vi "RX ADU.vi"(8 "error in (no error)":errorcluster, 9 "RX Data":string, 11 "MB_ADU_TCP in":refnum<class "MB_ADU_TCP.lvclass">) -> (0 "error out":errorcluster, 1 "PDU_resp":T1={"Function Code"=1, "Data"=[], "RTU_DataBytes"=0}, 3 "MB_ADU_TCP out":refnum<class "MB_ADU_TCP.lvclass">)   [LabVIEW 2016, in "MB Master.lvlib" / "MB_ADU_TCP.lvclass"]
doc: "Defines the receive procedure for a Modbus TCP ADU. The received PDU is written to PDU_resp."
uses:
  MB_ADU_TCP.lvclass
  MB_PDU/MB_PDU_Cluster.ctl
  MB Master.lvlib
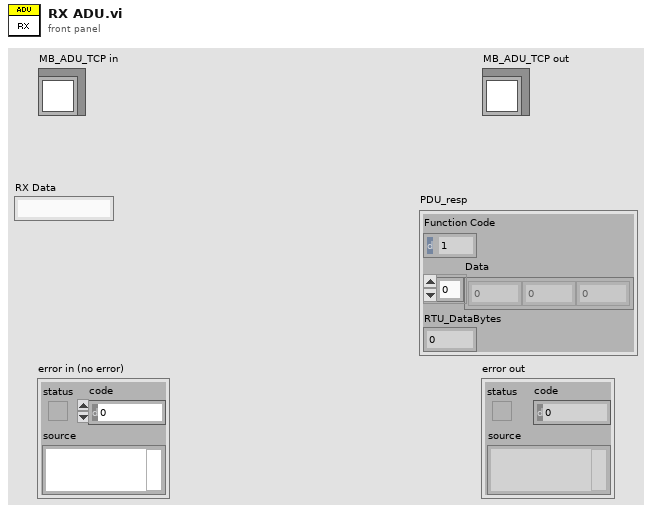
[diagram p1: front panel]
types:
  T1 = typedef "MB Master.lvlib/MB_PDU_Cluster.ctl" = cluster{"Function Code":u8, "Data":u8[], "RTU_DataBytes":i32}
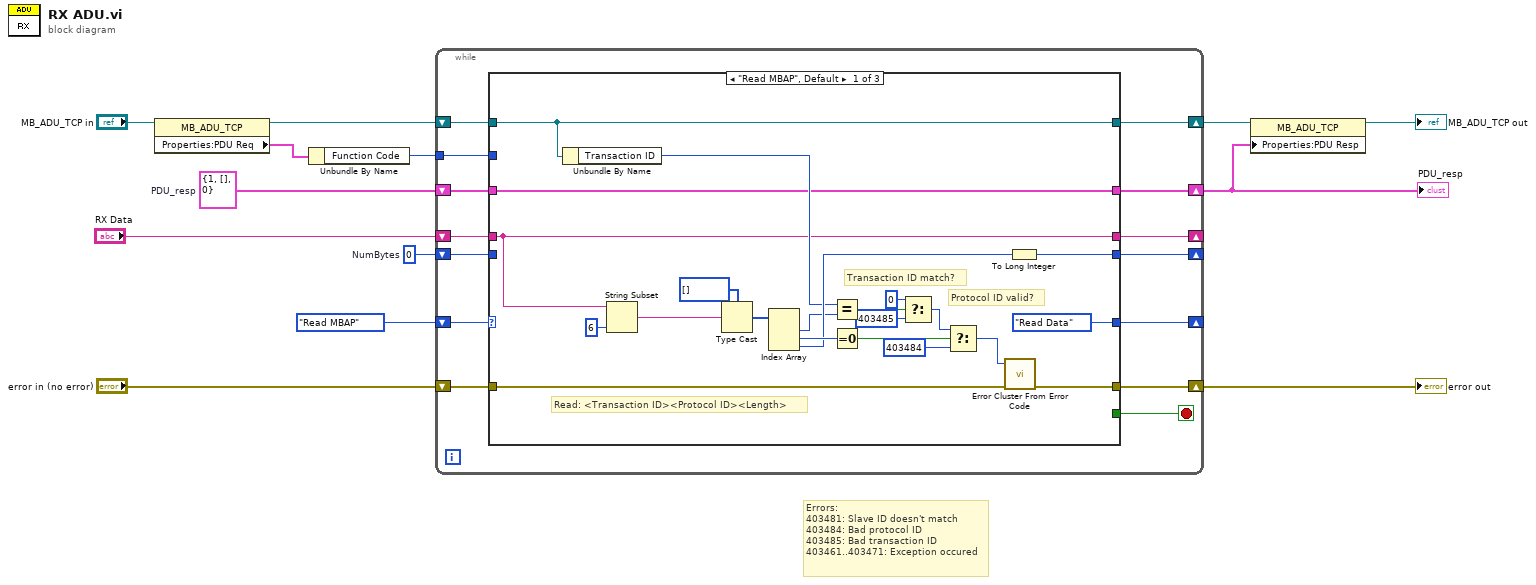
[diagram p0: block diagram]
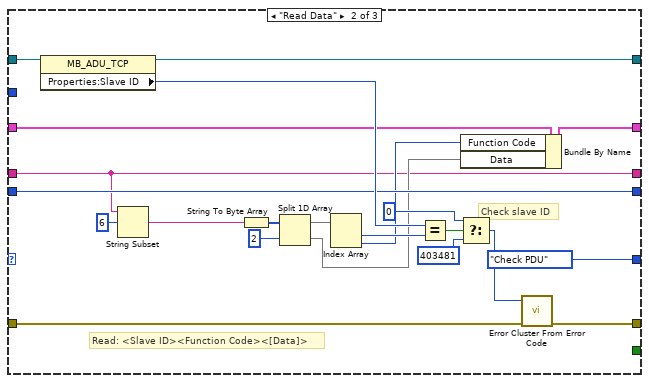
[diagram p2: hidden frame]
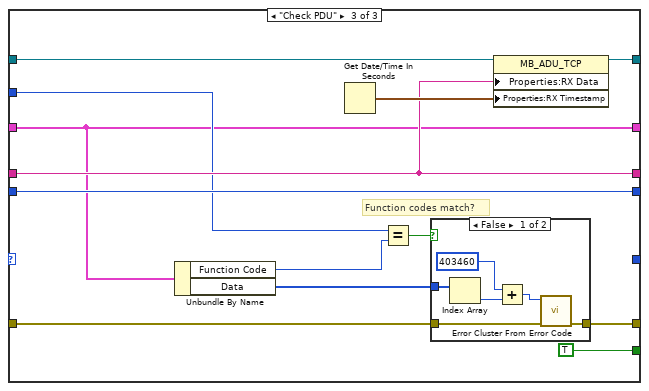
[diagram p3: hidden frame]
diagram:
  w7 = T1 {"Function Code"=1, "Data"=[], "RTU_DataBytes"=0}  # PDU_resp
  w10 = 0  # NumBytes
  # "Errors:\n403481: Slave ID doesn't match\n403484: Bad protocol ID\n403485: Bad transaction ID \n403461..403471: Exception occured"
  n1 = property class="MB_ADU_TCP"(reference="MB_ADU_TCP in") -> (reference out=w2:refnum<class "MB_ADU_TCP.lvclass">, "Properties:PDU Req"=w1:T1)  [unwired: 1 in, 1 out]
  n2 = Unbundle By Name(w1) -> ("Function Code"=w8:u8)
  n3 = while {
    shift-right: [w26] -> w11
    shift-left: "error in (no error)" -> [w25]
    shift-right: [w23] -> _
    shift-left: w10 -> [w20]
    shift-right: [w22] -> _
    shift-left: "RX Data" -> [w21]
    shift-right: [w18] -> w6
    shift-left: w2 -> [w19]
    shift-right: [w17] -> _
    shift-left: enum16{"Read MBAP", "Read Data", "Check PDU"}."Read MBAP" -> [w27]
    tunnel: w8 -> [w16]
    shift-right: [w14] -> w4
    shift-left: w7 -> [w15]
    stop <- w24 stop-if-true
    n4 = case shown="\"Read MBAP\", Default" w27 {
      tunnel: [w42 w61 w77] -> w26
      tunnel: w25 -> [w31 w51 w78]
      tunnel: [_ _ TRUE ("status")] -> w24
      tunnel: [w45 w59 w81] -> w23
      tunnel: [w29 w50 w82] -> w22
      tunnel: w21 -> [w29 w50 w82]
      tunnel: w20 -> [_ w59 w81]
      tunnel: w19 -> [w39 w60 w72]
      tunnel: [w39 w58 w83] -> w18
      tunnel: [enum16{"Read MBAP", "Read Data", "Check PDU"}."Read Data" enum16{"Read MBAP", "Read Data", "Check PDU"}."Check PDU" _] -> w17
      tunnel: w16 -> [_ _ w76]
      tunnel: w15 -> [w32 w57 w75]
      tunnel: [w32 w54 w75] -> w14
      frame "Read MBAP", Default {
        # "Transaction ID match?"
        # "Protocol ID valid?"
        # "Read: <Transaction ID><Protocol ID><Length>"
        n5 = Unbundle By Name(w39) -> ("Transaction ID"=w37:u16)
        n6 = String Subset(string=w29, length (rest)=6 ("length (rest)")) -> (substring=w28:string)  [unwired: 1 in]
        n7 = Type Cast(type=u16[] [], x=w28) -> (*(type *) &x=w48:u16[])
        n8 = Index Array(array=w48) -> (element #1=w38:u16, element #2=w47:u16, element #3=w46:u16)  [unwired: 3 in]
        n9 = Equal?(x=w37, y=w38) -> (x = y?=w36:bool)
        n10 = Equal To 0?(x=w47) -> (x = 0?=w44:bool)
        n11 = Select(t=0, s=w36, f=403485) -> (s? t:f=w34:i32)
        n12 = Select(t=w34, s=w44, f=403484) -> (s? t:f=w41:i32)
        n13 = call <vilib>:"Error Cluster From Error Code.vi"("error in (no error)"=w31, "error code (0)"=w41) -> ("error out"=w42:errorcluster)  [unwired: 7 in]
        n14 = To Long Integer(number=w46) -> (32bit integer=w45:i32)
      }
      frame "Read Data" {
        # "Check slave ID"
        # "Read: <Slave ID><Function Code><[Data]>"
        n15 = property class="MB_ADU_TCP"(reference=w60) -> (reference out=w58:refnum<class "MB_ADU_TCP.lvclass">, "Properties:Slave ID"=w66:u8)  [unwired: 1 in, 1 out]
        n16 = String Subset(string=w50, offset (0)=6) -> (substring=w52:string)  [unwired: 1 in]
        n17 = String To Byte Array(string=w52) -> (unsigned byte array=w71:u8[])
        n18 = Split 1D Array(array=w71, index=2) -> (first subarray=w70:u8[], second subarray=w55:u8[])
        n19 = Index Array(array=w70) -> (element #1=w67:u8, element #2=w56:u8)  [unwired: 2 in]
        n20 = Equal?(x=w66, y=w67) -> (x = y?=w65:bool)
        n21 = Bundle By Name(cluster=w57, "Function Code"=w56, "Data"=w55) -> (w54:T1)
        n22 = Select(t=0, s=w65, f=403481) -> (s? t:f=w62:i32)
        n23 = call <vilib>:"Error Cluster From Error Code.vi"("error in (no error)"=w51, "error code (0)"=w62) -> ("error out"=w61:errorcluster)  [unwired: 7 in]
      }
      frame "Check PDU" {
        # "Function codes match?"
        n24 = Unbundle By Name(w75) -> ("Function Code"=w74:u8, "Data"=w73:u8[])
        n25 = Get Date/Time In Seconds() -> (seconds since 1Jan1904=w84:timestamp)
        n26 = Equal?(x=w76, y=w74) -> (x = y?=w79:bool)
        n27 = case shown="False" w79 {
          tunnel: w73 -> [w89 _]
          tunnel: w78 -> [w87 w91]
          tunnel: [w86 w91] -> w77
          frame False {
            n28 = Index Array(array=w89) -> (element=w88:u8)  [unwired: 1 in]
            n29 = Add(x=403460 ("error code (0)"), y=w88) -> (x+y=w85:i32)
            n30 = call <vilib>:"Error Cluster From Error Code.vi"("error in (no error)"=w87, "error code (0)"=w85) -> ("error out"=w86:errorcluster)  [unwired: 7 in]
          }
          frame True {
          }
        }
        n31 = property class="MB_ADU_TCP"(reference=w72, "Properties:RX Data"=w82, "Properties:RX Timestamp"=w84) -> (reference out=w83:refnum<class "MB_ADU_TCP.lvclass">)  [unwired: 1 in, 1 out]
      }
    }
  }
  "error out" <- w11
  "PDU_resp" <- w4
  n32 = property class="MB_ADU_TCP"(reference=w6, "Properties:PDU Resp"=w4) -> (reference out=→"MB_ADU_TCP out":refnum<class "MB_ADU_TCP.lvclass">)  [unwired: 1 in, 1 out]
